vi "Glimpse set up to read sequence.vi"(0 "acquisition directory path":path, 3 "error in":errorcluster) -> (1 "Header2 file data out":T1, 4 "Header file data out":T2 {"Pixel depth" items=["8 bits", "16 bits", "Float", "Complex", "RGB", "HSL"]; "time of 1st frame, \nsec since 1/1/04" format="%.2f"}, 5 "acquisition directory path out":path=path "Glimpse set up to read sequence default value", 6 "Acquisition refnum array":refnum<file>[](array[refnum]), 7 "error out":errorcluster)   [LabVIEW 2015]
doc: "Opens the acquisition files and leaves them open. Opens the heaer file, reads it, and closes it. If there is an error, VI tries to close all open files before exiting."
uses:
  Header file data.ctl
  Seq file v 1/Offset table.ctl
  Seq file v 1/Offset.ctl
  Seq file v 1/file number.ctl
  Header2 file data.ctl
  GLIMPSE Globals.vi
panel:
  out "Number of acq files":i32
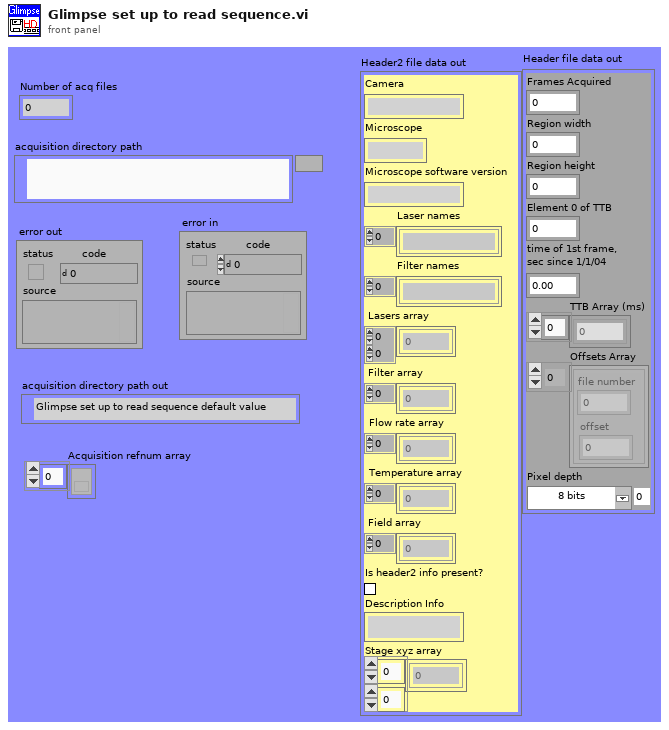
[diagram p1: front panel]
types:
  T1 = typedef "Header2 file data.ctl" = cluster{"Camera":string, "Microscope":string, "Microscope software version":string, "Laser names":string[], "Filter names":string[], "Lasers array":u16[][], "Filter array":u16[], "Flow rate array":dbl[], "Temperature array":dbl[], "Field array":u16[], "Is header2 info present?":bool, "Description Info":string, "Stage xyz array":dbl[][]}
  T2 = typedef "Header file data.ctl" = cluster{"Frames Acquired":u32, "Region width":i32, "Region height":i32, "Element 0 of TTB":u32, "time of 1st frame, \nsec since 1/1/04":dbl, "TTB Array (ms)":u32[], "Offsets Array":T3, "Pixel depth":u32}
  T3 = typedef "Offset table.ctl" = cluster{"offset":T4, "file number":T5}[]
  T4 = typedef "Offset.ctl" = i32
  T5 = typedef "file number.ctl" = u8
  T6 = enum16{"read/write", "read-only", "write-only", "write-only (truncate)"}
  T7 = enum16{"deny read/write", "deny write-only", "deny none"}
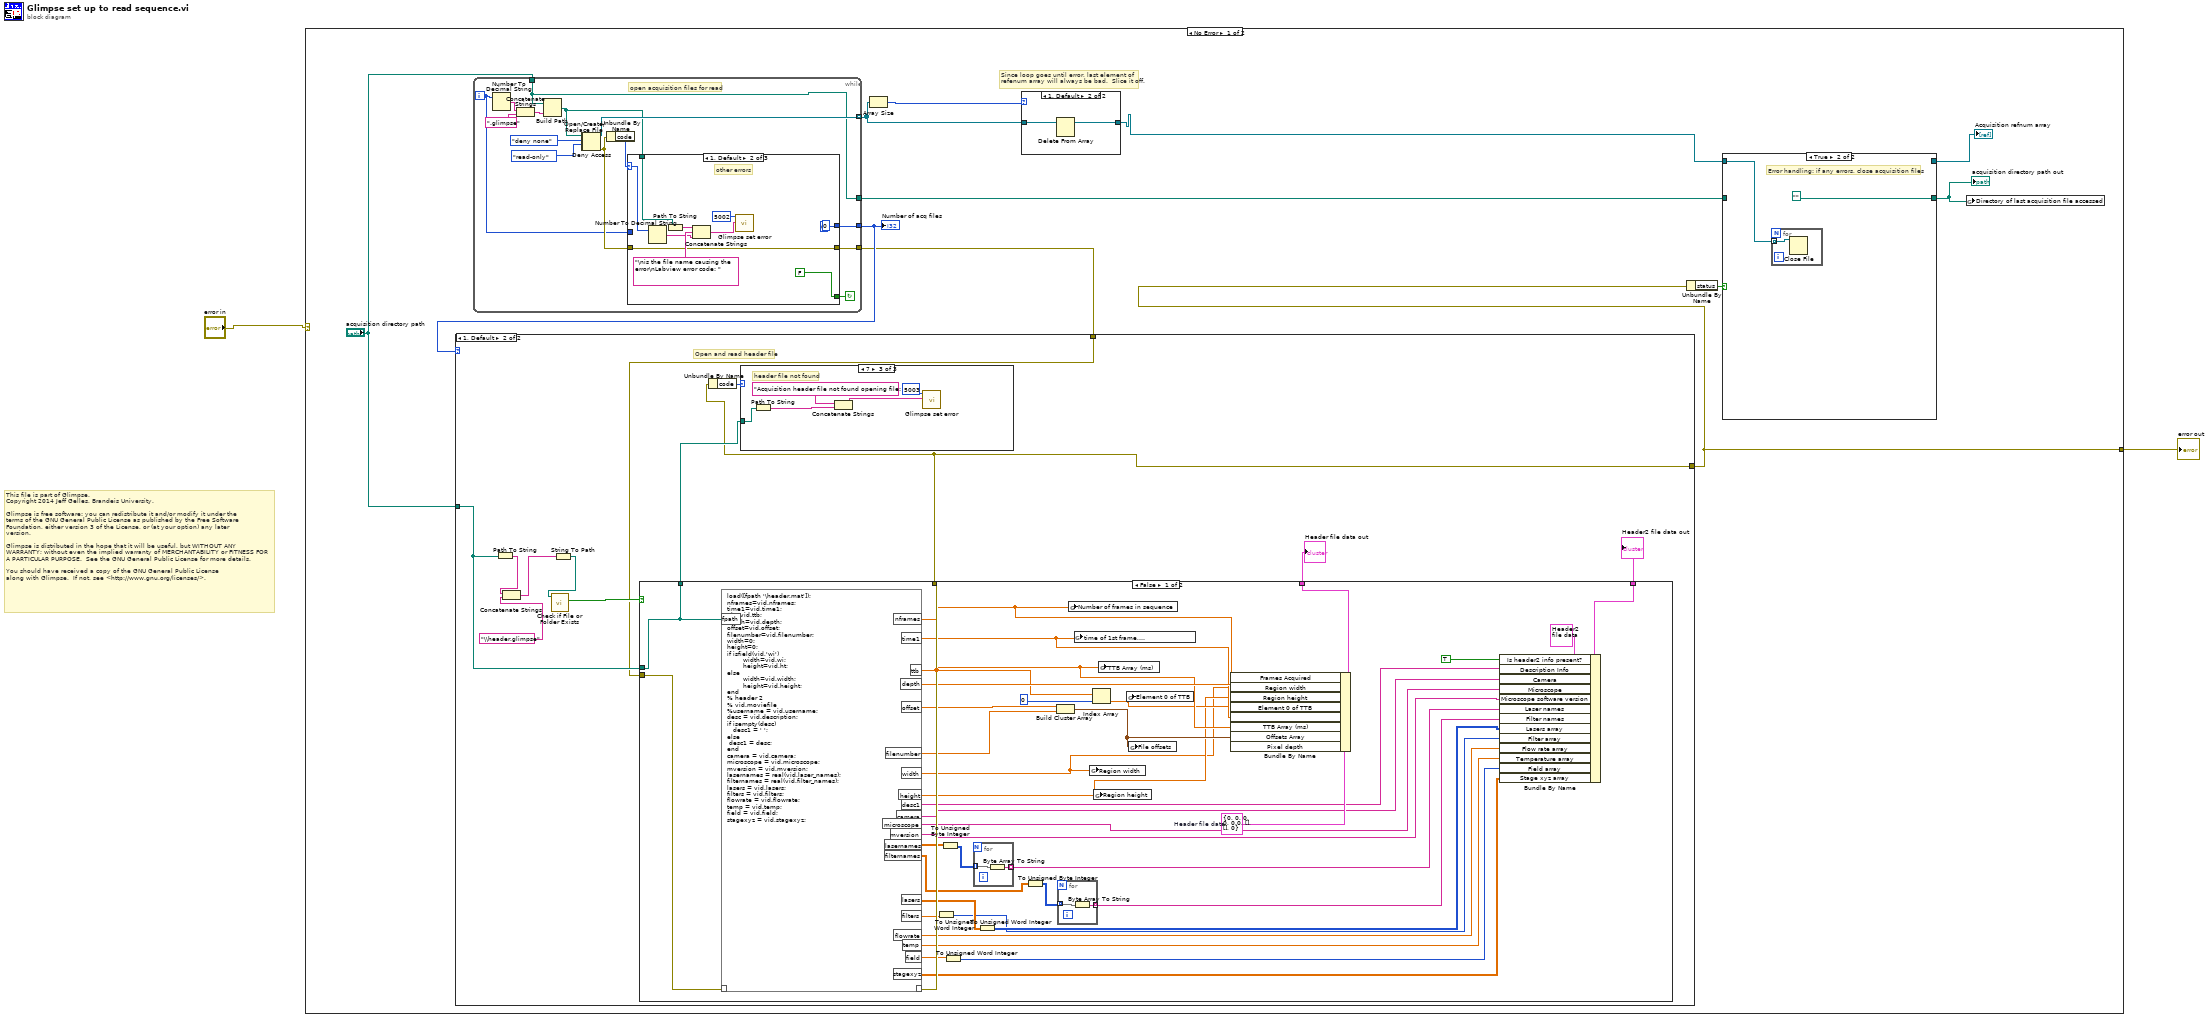
[diagram p0: block diagram]
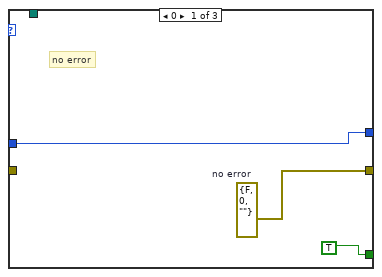
[diagram p3: hidden frame]
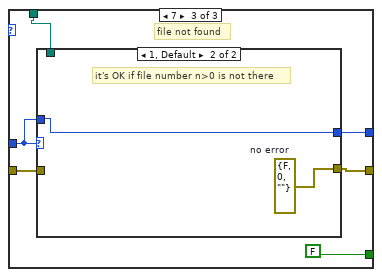
[diagram p4: hidden frame]
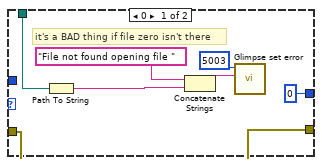
[diagram p5: hidden frame]
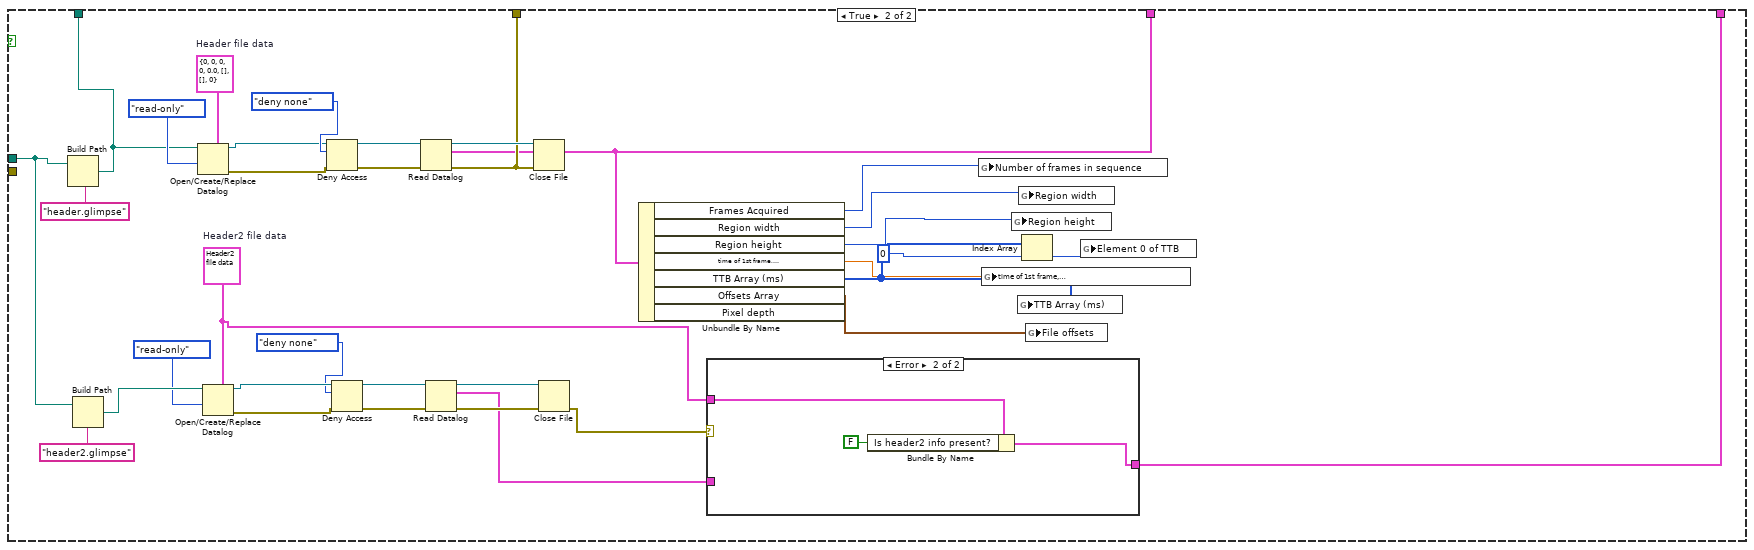
[diagram p7: hidden frame]
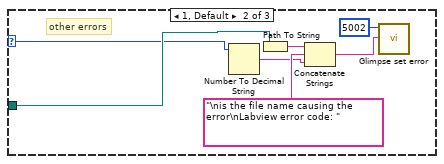
[diagram p10: hidden frame]
diagram:
  # "This file is part of Glimpse. \nCopyright 2014 Jeff Gelles, Brandeis University.    \n\nGlimpse is free software: you can redistribute it and/or modify it under the \nterms of the GNU General Public License as published by the Free Software \nFoundation, either version 3 of the License, or (at your option) any later \nversion.\n\nGlimpse is distributed in the hope that it will be useful, but WITHOUT ANY \nWARRANTY; without even the implied warranty of MERCHANTABILITY or FITNESS FOR \nA PARTICULAR PURPOSE.  See the GNU General Public License for more details.\n\nYou should have received a copy of the GNU General Public License\nalong with Glimpse.  If not, see <http://www.gnu.org/licenses/>."
  n1 = case shown="No Error" "error in" {
    selector: "error in" -> [_ w172]
    tunnel: [w4 w172] -> w2
    frame No Error {
      # "Since loop goes until error, last element of\nrefenum array will always be bad.  Slice it off."
      n2 = while {
        tunnel: "acquisition directory path" -> [w19]
        tunnel: [w19] -> w8
        tunnel: [w24] -> w13
        tunnel: [w22] -> w9 mode=indexing
        tunnel: [w21] -> w12
        i -> [w25]
        stop <- w23 continue-if-true
        # "open acquisition files for read"
        n3 = Number To Decimal String(number=w25) -> (decimal integer string=w32:string)  [unwired: 1 out]
        n4 = Concatenate Strings(w32, ".glimpse" ("string")) -> (w30:string)
        n5 = Build Path(base path=w19, name or relative path=w30) -> (appended path=w20:path)
        n6 = Open/Create/Replace File(file path (use dialog)=w20, access (0:read/write)=T6."read-only" ("open mode (0)")) -> (refnum out=w17:refnum<file>, error out=w18:errorcluster)  [unwired: 1 in, 4 out]
        n7 = Deny Access(4:w18, 6:T7."deny none" ("deny mode (2)"), 7:w17) -> (0:w26:errorcluster, 3:w22:refnum<file>)
        n8 = Unbundle By Name(w26) -> ("code"=w27:i32)
        n9 = case shown="1, Default" w27 {
          selector: w27 -> [_ w36 _]
          tunnel: w26 -> [_ w40 w47]
          tunnel: w20 -> [_ w45 w49]
          tunnel: w25 -> [w35 _ w51]
          tunnel: [w35 0 w50] -> w24
          tunnel: [TRUE FALSE FALSE] -> w23
          tunnel: [w33 w40 w46] -> w21
          frame 0 {
            w33 = errorcluster {"status"=FALSE, "code"=0, "source"=""}  # no error
            # "no error"
          }
          frame 1, Default {
            (unwired) 0
            # "other errors"
            n10 = Number To Decimal String(number=w36) -> (decimal integer string=w38:string)  [unwired: 1 out]
            n11 = Path To String(path=w45) -> (string=w42:string)
            n12 = Concatenate Strings(w42, "\nis the file name causing the error\nLabview error code: " ("string"), w38) -> (w37:string)
            n13 = call "Glimpse set error.vi"("code"=5002, "Additional information"=w37) -> ()  [unwired: 1 in, 6 out]
          }
          frame 7 {
            # "file not found"
            n14 = case shown="1, Default" w51 {
              tunnel: w51 -> [_ w60]
              tunnel: [0 w60] -> w50
              tunnel: w49 -> [w55 _]
              tunnel: [w54 w59] -> w46
              tunnel: w47 -> [w54 _]
              frame 0 {
                # "it's a BAD thing if file zero isn't there"
                n15 = Path To String(path=w55) -> (string=w57:string)
                n16 = Concatenate Strings("File not found opening file " ("string"), w57) -> (w52:string)
                n17 = call "Glimpse set error.vi"("code"=5003, "Additional information"=w52) -> ()  [unwired: 1 in, 6 out]
              }
              frame 1, Default {
                w59 = errorcluster {"status"=FALSE, "code"=0, "source"=""}  # no error
                # "it's OK if file number n>0 is not there"
              }
            }
          }
        }
      }
      "Number of acq files" <- w13
      n18 = case shown="1, Default" w13 {
        tunnel: [w61 w64] -> w4
        tunnel: w12 -> [w61 w65]
        tunnel: "acquisition directory path" -> [_ w67]
        frame 0 {
        }
        frame 1, Default {
          # "Open and read header file"
          n19 = Path To String(path=w67) -> (string=w71:string)
          n20 = Concatenate Strings(w71, "\\header.glimpse" ("search string")) -> (w69:string)
          n21 = String To Path(string=w69) -> (path=w72:path)
          n22 = call <vilib>:"Check if File or Folder Exists.vi"("path"=w72) -> ("file or folder exists?"=w68:bool)  [unwired: 1 in, 9 out]
          n23 = case shown="False" w68 {
            tunnel: w67 -> [w108 w120]
            tunnel: [w108 w147] -> w66
            tunnel: w65 -> [w110 _]
            tunnel: [w109 w134] -> w64
            tunnel: [w106 w131] -> w63
            tunnel: [w93 w116] -> w62
            frame False {
              w107 = T2 {"Frames Acquired"=0, "Region width"=0, "Region height"=0, "Element 0 of TTB"=0, "time of 1st frame, \nsec since 1/1/04"=0.0, "TTB Array (ms)"=[], "Offsets Array"=[], "Pixel depth"=0}  # Header file data
              n24 = script code="load([fpath '\\header.mat']);\nnframes=vid.nframes;\ntime1=vid.time1;\nttb=vid.ttb;\ndepth=vid.depth;\noffset=vid.offset;\nfilenumber=vid.filenumber;\nwidth=0;\nheight=0;\nif isfield(vid,'wi')\n        width=vid.wi;\n        height=vid.ht;\nelse\n        width=vid.width;\n        height=vid.height;\nend\n% header 2\n% vid.moviefile\n%username = vid.username;\ndesc = vid.description;\nif isempty(desc)\n   desc1 = ' ';\nelse\n desc1 = desc;\nend\ncamera = vid.camera;\nmicroscope = vid.microscope;\nmversion = vid.mversion;\nlasernames = real(vid.laser_names);\nfilternames = real(vid.filter_names);\nlasers = vid.lasers;\nfilters = vid.filters;\nflowrate = vid.flowrate;\ntemp = vid.temp;\nfield = vid.field;\nstagexyz = vid.stagexyz;"("??"=w110, "fpath"=w108) -> ("??"=w109:errorcluster, "nframes"=w98:dbl, "time1"=w102:dbl, "ttb"=w103:dbl[], "offset"=w96:dbl[], "filenumber"=w97:dbl[], "width"=w99:dbl, "height"=w100:dbl, "depth"=w105:dbl, "desc1"=w92:string, "camera"=w91:string, "microscope"=w90:string, "mversion"=w89:string, "lasernames"=w88:dbl[][], "filternames"=w84:dbl[][], "lasers"=w82:dbl[][], "filters"=w80:dbl[], "flowrate"=w78:dbl[], "temp"=w77:dbl[], "field"=w76:dbl[], "stagexyz"=w74:dbl[][])
              n25 = To Unsigned Word Integer(number=w80) -> (unsigned 16bit integer=w79:u16[])
              n26 = To Unsigned Byte Integer(number=w88) -> (unsigned 8bit integer=w87:u8[][])
              n27 = To Unsigned Word Integer(number=w76) -> (unsigned 16bit integer=w75:u16[])
              n28 = for {
                tunnel: w87 -> [w115] mode=indexing
                tunnel: [w114] -> w86 mode=indexing
                n29 = Byte Array To String(unsigned byte array=w115) -> (string=w114:string)
              }
              n30 = To Unsigned Word Integer(number=w82) -> (unsigned 16bit integer=w81:u16[][])
              n31 = To Unsigned Byte Integer(number=w84) -> (unsigned 8bit integer=w85:u8[][])
              n32 = Build Cluster Array(w96, w97) -> (w104:cluster{dbl, dbl}[])
              n33 = for {
                tunnel: w85 -> [w113] mode=indexing
                tunnel: [w112] -> w83 mode=indexing
                n34 = Byte Array To String(unsigned byte array=w113) -> (string=w112:string)
              }
              n35 = global write "GLIMPSE Globals.vi" "Number of frames in sequence"(w98) -> ()
              n36 = global write "GLIMPSE Globals.vi" "time of 1st frame, \nsec since 1/1/04"(w102) -> ()
              n37 = global write "GLIMPSE Globals.vi" "Region width"(w99) -> ()
              n38 = Index Array(array=w103, index=0) -> (element=w101:dbl)
              n39 = global write "GLIMPSE Globals.vi" "Region height"(w100) -> ()
              n40 = global write "GLIMPSE Globals.vi" "TTB Array (ms)"(w103) -> ()
              n41 = global write "GLIMPSE Globals.vi" "Element 0 of TTB"(w101) -> ()
              n42 = global write "GLIMPSE Globals.vi" "File offsets"(w104) -> ()
              n43 = Bundle By Name(cluster=w107, "Frames Acquired"=w98, "Region width"=w99, "Region height"=w100, "Element 0 of TTB"=w101, "time of 1st frame, \nsec since 1/1/04"=w102, "TTB Array (ms)"=w103, "Offsets Array"=w104, "Pixel depth"=w105) -> (w106:T2)
              n44 = Bundle By Name(cluster=T1 {"Camera"="", "Microscope"="", "Microscope software version"="", "Laser names"=[], "Filter names"=[], "Lasers array"=[], "Filter array"=[], "Flow rate array"=[], "Temperature array"=[], "Field array"=[], "Is header2 info present?"=FALSE, "Description Info"="", "Stage xyz array"=[]} ("input cluster"), "Is header2 info present?"=TRUE, "Description Info"=w92, "Camera"=w91, "Microscope"=w90, "Microscope software version"=w89, "Laser names"=w86, "Filter names"=w83, "Lasers array"=w81, "Filter array"=w79, "Flow rate array"=w78, "Temperature array"=w77, "Field array"=w75, "Stage xyz array"=w74) -> (w93:T1)
            }
            frame True {
              w117 = T1 {"Camera"="", "Microscope"="", "Microscope software version"="", "Laser names"=[], "Filter names"=[], "Lasers array"=[], "Filter array"=[], "Flow rate array"=[], "Temperature array"=[], "Field array"=[], "Is header2 info present?"=FALSE, "Description Info"="", "Stage xyz array"=[]}  # Header2 file data
              w149 = T2 {"Frames Acquired"=0, "Region width"=0, "Region height"=0, "Element 0 of TTB"=0, "time of 1st frame, \nsec since 1/1/04"=0.0, "TTB Array (ms)"=[], "Offsets Array"=[], "Pixel depth"=0}  # Header file data
              n45 = Build Path(base path=w120, name or relative path="header.glimpse" ("search string")) -> (appended path=w147:path)
              n46 = Build Path(base path=w120, name or relative path="header2.glimpse" ("search string")) -> (appended path=w123:path)
              n47 = Open/Create/Replace Datalog(5:w149, 9:T6."read-only" ("open mode (0)"), 11:w147) -> (0:w132:errorcluster, 3:w133:refnum<k1>)  [unwired: 1 in, 3 out]
              n48 = Open/Create/Replace Datalog(5:w117, 9:T6."read-only" ("open mode (0)"), 11:w123) -> (0:w130:errorcluster, 3:w129:refnum<k1>)  [unwired: 1 in, 3 out]
              n49 = Deny Access(4:w132, 6:T7."deny none" ("deny mode (2)"), 7:w133) -> (0:w145:errorcluster, 3:w144:refnum<k1>)
              n50 = Deny Access(4:w130, 6:T7."deny none" ("deny mode (2)"), 7:w129) -> (0:w125:errorcluster, 3:w126:refnum<k1>)
              n51 = Read Datalog(4:w145, 7:w144) -> (0:w134:errorcluster, 2:w131:T2, 3:w143:refnum<k1>)  [unwired: 1 out]
              n52 = Read Datalog(4:w125, 7:w126) -> (0:w128:errorcluster, 2:w118:T1, 3:w127:refnum<k1>)  [unwired: 1 out]
              n53 = Close File(refnum=w143, error in=w134) -> ()  [unwired: 2 out]
              n54 = Close File(refnum=w127, error in=w128) -> (error out=w119:errorcluster)  [unwired: 1 out]
              n55 = Unbundle By Name(w131) -> ("Frames Acquired"=w142:u32, "Region width"=w141:i32, "Region height"=w140:i32, "time of 1st frame, \nsec since 1/1/04"=w139:dbl, "TTB Array (ms)"=w136:u32[], "Offsets Array"=w138:T3)  [unwired: 1 out]
              n56 = case shown="Error" w119 {
                tunnel: w118 -> [w151 _]
                tunnel: w117 -> [_ w154]
                tunnel: [w151 w153] -> w116
                frame No Error {
                }
                frame Error {
                  n57 = Bundle By Name(cluster=w154, "Is header2 info present?"=FALSE) -> (w153:T1)
                }
              }
              n58 = global write "GLIMPSE Globals.vi" "Number of frames in sequence"(w142) -> ()
              n59 = global write "GLIMPSE Globals.vi" "time of 1st frame, \nsec since 1/1/04"(w139) -> ()
              n60 = global write "GLIMPSE Globals.vi" "Region height"(w140) -> ()
              n61 = global write "GLIMPSE Globals.vi" "TTB Array (ms)"(w136) -> ()
              n62 = global write "GLIMPSE Globals.vi" "Region width"(w141) -> ()
              n63 = Index Array(array=w136, index=0) -> (element=w137:u32)
              n64 = global write "GLIMPSE Globals.vi" "File offsets"(w138) -> ()
              n65 = global write "GLIMPSE Globals.vi" "Element 0 of TTB"(w137) -> ()
            }
          }
          "Header file data out" <- w63
          "Header2 file data out" <- w62
          n66 = Unbundle By Name(w64) -> ("code"=w73:i32)
          n67 = case shown="7" w73 {
            selector: w73 -> [_ w155 _]
            tunnel: w66 -> [_ w156 w164]
            frame 0 {
              # "no error"
            }
            frame 1, Default {
              # "other errors"
              n68 = Number To Decimal String(number=w155) -> (decimal integer string=w158:string)  [unwired: 1 out]
              n69 = Path To String(path=w156) -> (string=w161:string)
              n70 = Concatenate Strings(w161, "\nis the file name causing the error\nLabview error code: " ("string"), w158) -> (w157:string)
              n71 = call "Glimpse set error.vi"("code"=5002, "Additional information"=w157) -> ()  [unwired: 1 in, 6 out]
            }
            frame 7 {
              # "header file not found"
              n72 = Path To String(path=w164) -> (string=w165:string)
              n73 = Concatenate Strings("Acquisition header file not found opening file: " ("string"), w165) -> (w162:string)
              n74 = call "Glimpse set error.vi"("code"=5003, "Additional information"=w162) -> ()  [unwired: 1 in, 6 out]
            }
          }
        }
      }
      n75 = Array Size(array=w9) -> (size(s)=w10:i32)
      n76 = case shown="1, Default" w10 {
        tunnel: w9 -> [w14 w16]
        tunnel: [w14 w15] -> w5
        frame 0 {
        }
        frame 1, Default {
          n77 = Delete From Array(array=w16) -> (array with subset deleted=w15:refnum<file>[])  [unwired: 2 in, 1 out]
        }
      }
      n78 = Unbundle By Name(w4) -> ("status"=w3:bool)
      n79 = case shown="True" w3 {
        tunnel: w8 -> [w168 _]
        tunnel: [w168 path ""] -> w7
        tunnel: [w167 _] -> w6
        tunnel: w5 -> [w167 w169]
        frame False {
          # "no errors"
        }
        frame True {
          # "Error handling: if any errors, close acquisition files"
          n80 = for {
            tunnel: w169 -> [w171] mode=indexing
            n81 = Close File(refnum=w171) -> ()  [unwired: 1 in, 2 out]
          }
        }
      }
      "acquisition directory path out" <- w7
      "Acquisition refnum array" <- w6
      n82 = global write "GLIMPSE Globals.vi" "Directory of last acquisition file accessed"(w7) -> ()
    }
    frame Error {
    }
  }
  "error out" <- w2
